vi "Get JoyStick 2014.vi"() -> (3 "input cluster":T1)   [LabVIEW 2014]
uses:
  Controls.ctl
  Global Variables/Refnums.vi
  <vilib>/Rock Robotics/WPI/Joystick/WPI_JoystickGetSetRefNum.vi
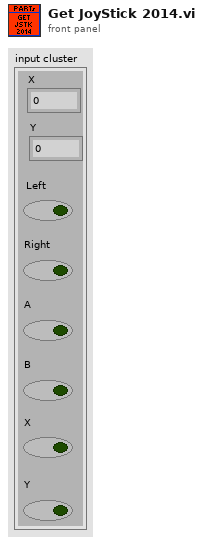
[diagram p1: front panel]
types:
  T1 = typedef "Controls.ctl" = cluster{"X":dbl, "Y":dbl, "Left":bool, "Right":bool, "A":bool, "B":bool, "X":bool, "Y":bool}
  T2 = typedef "WPI_JoystickDevRef.ctl" = cluster{"Device":T3}
  T3 = typedef "WPI_JoystickDeviceEnum.ctl" = enum16{"USB 0", "USB 1", "USB 2", "USB 3", "USB 4", "USB 5"}
  T4 = cluster{"Axes[0]":dbl, "Axes[1]":dbl, "Axes[2]":dbl, "Axes[3]":dbl, "Axes[4]":dbl, "Axes[5]":dbl, "Axes[6]":dbl, "Axes[7]":dbl, "Axes[8]":dbl}
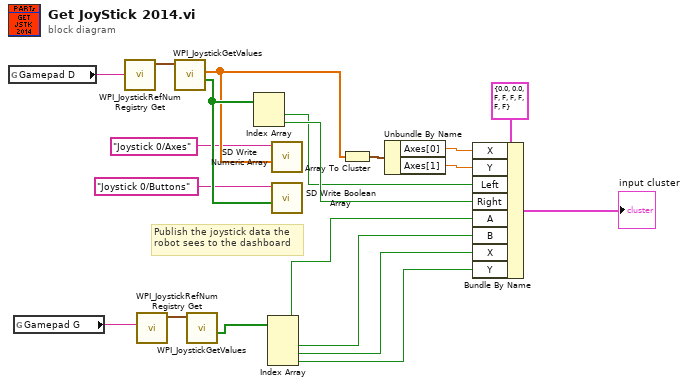
[diagram p0: block diagram]
diagram:
  # "Publish the joystick data the\nrobot sees to the dashboard"
  n1 = global read "Refnums.vi" "Gamepad D"() -> (w5:string)
  n2 = global read "Refnums.vi" "Gamepad G"() -> (w6:string)
  n3 = call <vilib>:"WPI_JoystickRefNum Registry Get.vi"("refnum name"=w5) -> ("JoystickDevRef"=w4:T2)  [unwired: 1 in, 9 out]
  n4 = call <vilib>:"WPI_JoystickRefNum Registry Get.vi"("refnum name"=w6) -> ("JoystickDevRef"=w1:T2)  [unwired: 1 in, 9 out]
  n5 = call <vilib>:"WPI_JoystickGetValues.vi"("JoystickDevRef"=w4) -> ("Buttons"=w11:bool[], "Axes"=w7:dbl[])  [unwired: 6 in, 3 out]
  n6 = call <vilib>:"WPI_JoystickGetValues.vi"("JoystickDevRef"=w1) -> ("Buttons"=w14:bool[])  [unwired: 6 in, 4 out]
  n7 = Index Array(array=w11) -> (element #1=w12:bool, element #2=w13:bool)  [unwired: 2 in]
  n8 = Index Array(array=w14) -> (element #1=w15:bool, element #2=w16:bool, element #3=w17:bool, element #4=w18:bool)  [unwired: 4 in]
  n9 = call <vilib>:"SD Write Numeric Array.vi"("Numeric Array"=w7, "Name"="Joystick 0/Axes") -> ()  [unwired: 8 in, 2 out]
  n10 = call <vilib>:"SD Write Boolean Array.vi"("Boolean Array"=w11, "Name"="Joystick 0/Buttons") -> ()  [unwired: 8 in, 2 out]
  n11 = Array To Cluster(array=w7) -> (cluster=w8:T4)
  n12 = Unbundle By Name(w8) -> ("Axes[0]"=w9:dbl, "Axes[1]"=w10:dbl)
  n13 = Bundle By Name(cluster=T1 {"X"=0.0, "Y"=0.0, "Left"=FALSE, "Right"=FALSE, "A"=FALSE, "B"=FALSE, "X"=FALSE, "Y"=FALSE} ("input cluster"), "X"=w9, "Y"=w10, "Left"=w12, "Right"=w13, "A"=w15, "B"=w16, "X"=w17, "Y"=w18) -> (→"input cluster":T1)
